vi "get_component_type_name.vi"(8 "error in (no error)":errorcluster, 11 "GenericInstrument in":refnum<class "GenericInstrument.lvclass">) -> (0 "error out":errorcluster, 2 "component type":string, 3 "GenericInstrument out":refnum<class "GenericInstrument.lvclass">)   [LabVIEW 2010, in "GenericInstrument.lvclass"]
uses:
  GenericInstrument.lvclass
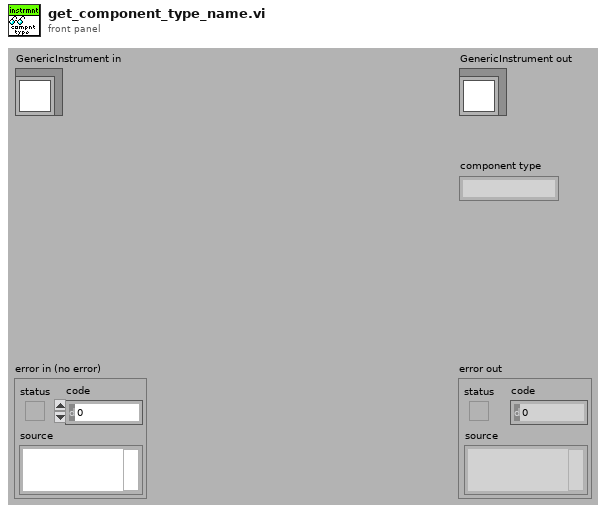
[diagram p1: front panel]
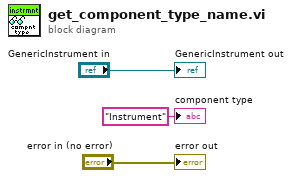
[diagram p0: block diagram]
diagram:
  "error out" <- "error in (no error)"
  "GenericInstrument out" <- "GenericInstrument in"
  "component type" <- "Instrument" ("component type")
